vi "Create Observer Registry.vi"(8 "error in (no error)":errorcluster) -> (0 "error out":errorcluster, 3 "ObsReg":refnum<class "ObserverRegistry.lvclass">)   [LabVIEW 2011, in "Messenging.lvlib" / "ObserverRegistry.lvclass"]
doc: "A registry of messages that can be observed and observers of these messages. Observer processes can register by sending registration messages (command pattern) that are acted on by \"Register.vi\". Messages to be observed are posted by \"Notify Observers\" VI's, which comes in two types: \"Events\" are posted to any registered observer; \"State\" is posted only if it has changed, and is stored by the registry so that any new Observer can be immediately informed of the current state.\n\nSee the \"Parallel Process\" examples for use of the Registry.\n\nNote that the Registry is a by-ref object, and thus a single Registry can be shared across multiple loops."
uses:
  ObserverRegistry.lvclass
  ObserverRegistry.lvclass/ObserverRegistry.ctl
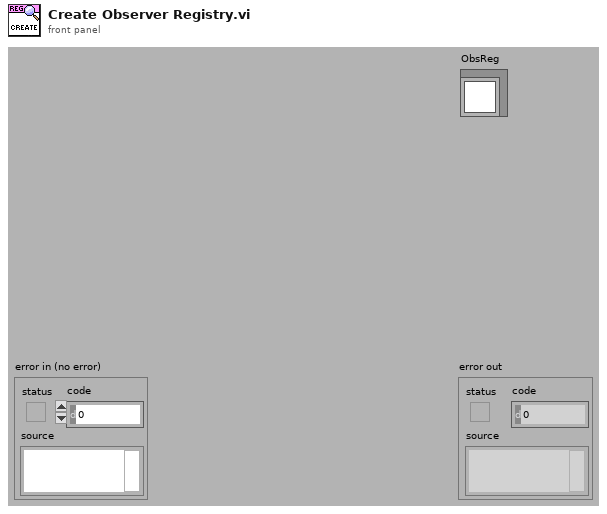
[diagram p1: front panel]
types:
  T1 = typedef "Messenging.lvlib/ObserverRegistry.lvclass/ObserverRegistryData.ctl" = cluster{"Observer of Errors":refnum<class "Observer.lvclass">, "Observer of All":refnum<class "Observer.lvclass">, "Event Registry":variant}
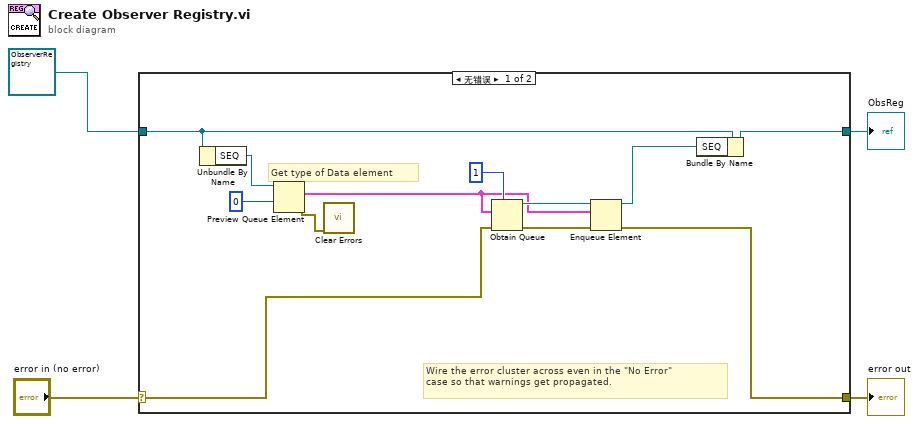
[diagram p0: block diagram]
diagram:
  n1 = case shown="无错误" "error in (no error)" {
    selector: "error in (no error)" -> [w9 w18]
    tunnel: [w6 w18] -> w3
    tunnel: [w15 w17] -> w1
    tunnel: refnum<class "ObserverRegistry.lvclass"> refnum ("ObserverRegistry in") -> [w13 w17]
    frame No Error {
      # "Get type of Data element"
      # "Wire the error cluster across even in the \"No Error\"\ncase so that warnings get propagated."
      n2 = Unbundle By Name(w13) -> ("SEQ"=w12:refnum<queue>)
      n3 = Preview Queue Element(queue=w12, timeout in ms (-1)=0) -> (element=w5:T1, error out=w10:errorcluster)  [unwired: 1 in, 2 out]
      n4 = call <vilib>:"Clear Errors.vi"("error in (no error)"=w10) -> ()  [unwired: 7 out]
      n5 = Obtain Queue(max queue size (-1, unlimited)=1, element data type=w5, error in (no error)=w9) -> (queue out=w14:refnum<queue>, error out=w7:errorcluster)  [unwired: 1 in, 2 out]
      n6 = Enqueue Element(queue=w14, element=w5, error in (no error)=w7) -> (queue out=w8:refnum<queue>, error out=w6:errorcluster)  [unwired: 2 out]
      n7 = Bundle By Name(cluster=w13, "SEQ"=w8) -> (w15:refnum<class "ObserverRegistry.lvclass">)
    }
    frame Error {
    }
  }
  "error out" <- w3
  "ObsReg" <- w1
